vi "set_triggered.vi"(8 "error in (no error)":errorcluster, 10 "triggered?":bool, 11 "DL090202ScanHead.lvclass in":refnum<class "ScanHeadDL090202.lvclass">) -> (0 "error out":errorcluster, 3 "DL090202ScanHead.lvclass out":refnum<class "ScanHeadDL090202.lvclass">)   [LabVIEW 2010, in "ScanHeadDL090202.lvclass"]
uses:
  ScanHeadDL090202.lvclass
  ScanHeadDL090202.lvclass/ScanHeadDL090202.ctl
  Clock/GenericClock/GenericClock/GenericClock.lvclass
  GenericScanHead/GenericScanHead/GenericScanHead.lvclass
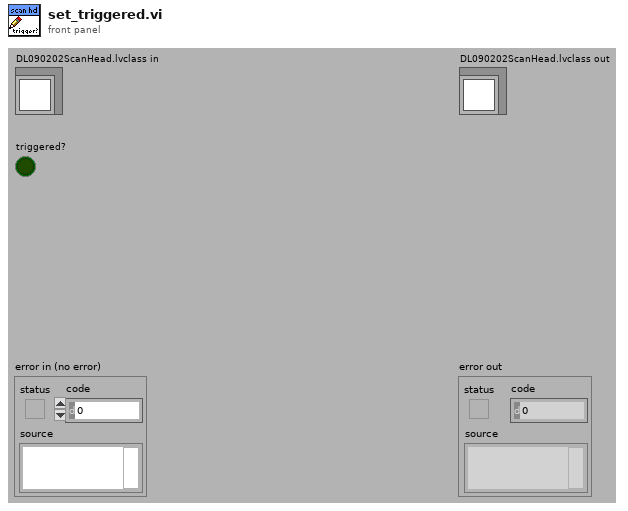
[diagram p1: front panel]
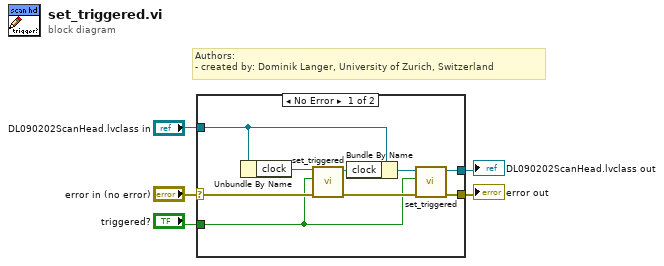
[diagram p0: block diagram]
diagram:
  # "Authors: \n- created by: Dominik Langer, University of Zurich, Switzerland"
  n1 = case shown="No Error" "error in (no error)" {
    selector: "error in (no error)" -> [w12 w15]
    tunnel: [w14 w15] -> w5
    tunnel: [w13 w16] -> w4
    tunnel: "triggered?" -> [w9 _]
    tunnel: "DL090202ScanHead.lvclass in" -> [w7 w16]
    frame No Error {
      n2 = Unbundle By Name(w7) -> ("clock"=w10:refnum<class "GenericClock.lvclass">)
      n3 = call-dynamic "set_triggered.vi"("error in (no error)"=w12, "triggered?"=w9, "GenericClock.lvclass in"=w10) -> ("error out"=w11:errorcluster, "GenericClock.lvclass out"=w8:refnum<class "GenericClock.lvclass">)  [unwired: 7 out]
      n4 = Bundle By Name(cluster=w7, "clock"=w8) -> (w6:refnum<class "ScanHeadDL090202.lvclass">)
      n5 = call-parent "set_triggered.vi"("error in (no error)"=w11, "triggered?"=w9, "GenericScanHead.lvclass in"=w6) -> ("error out"=w14:errorcluster, "GenericScanHead.lvclass out"=w13:refnum<class "ScanHeadDL090202.lvclass">)  [unwired: 7 out]
    }
    frame Error {
    }
  }
  "error out" <- w5
  "DL090202ScanHead.lvclass out" <- w4
